vi "test_find_shift.vi"() -> ()   [LabVIEW 2016]
uses:
  <vilib>/Platform/TimedLoop/XDataNode/timing_clust.ctl
  <vilib>/Platform/TimedLoop/XDataNode/nitl_modes.ctl
  <vilib>/Platform/TimedLoop/XDataNode/wakeup.ctl
  <vilib>/platform/TimedLoop/XDataNode/XDataNode.xnode
  <vilib>/Platform/TimedLoop/XDataNode/XDNodeRunTimeDep.lvlib
panel:
  out "Ref Cropped":T1(plugin-control)
  out "ROI":T1(plugin-control)
  out "Y Pos":i32[](array[numeric])
  out "X Pos":i32[](array[numeric])
  out "Y Pos":i32[](graph)
  out "X Pos":i32[](graph)
  out "Surface Height":dbl[](graph)
  out "Y Shift":i32[](graph)
  out "X Shift":i32[](graph)
  out "Current Image":dbl=1000.0
  out "Surface Height":i32[](array[numeric])
  out "Y Shifts":i32[](array[numeric])
  out "X Shifts":i32[](array[numeric])
  in  "Vertical Search Range":dbl=50.0
  in  "ROI Horizontal Size":dbl=50.0
  in  "ROI Vertical Size":dbl=50.0
  in  "ROI Vertical Offset":dbl
  in  "Struc El Size":i32=10
  in  "Threshold Multiplier":sgl=2.0
  in  "Simulated FPS":dbl=50.0
  in  "stop":bool
  out "Num Images":dbl=1000.0
  in  "AVI File for Simulated Raw B Scan Images":path=path "C:/Users/Applied Optics Group/Desktop/DCF Paper Data Processing/data/2020_08_04_2dcheckerboard_AF/Large_grid/OCT_raw_vol.avi"
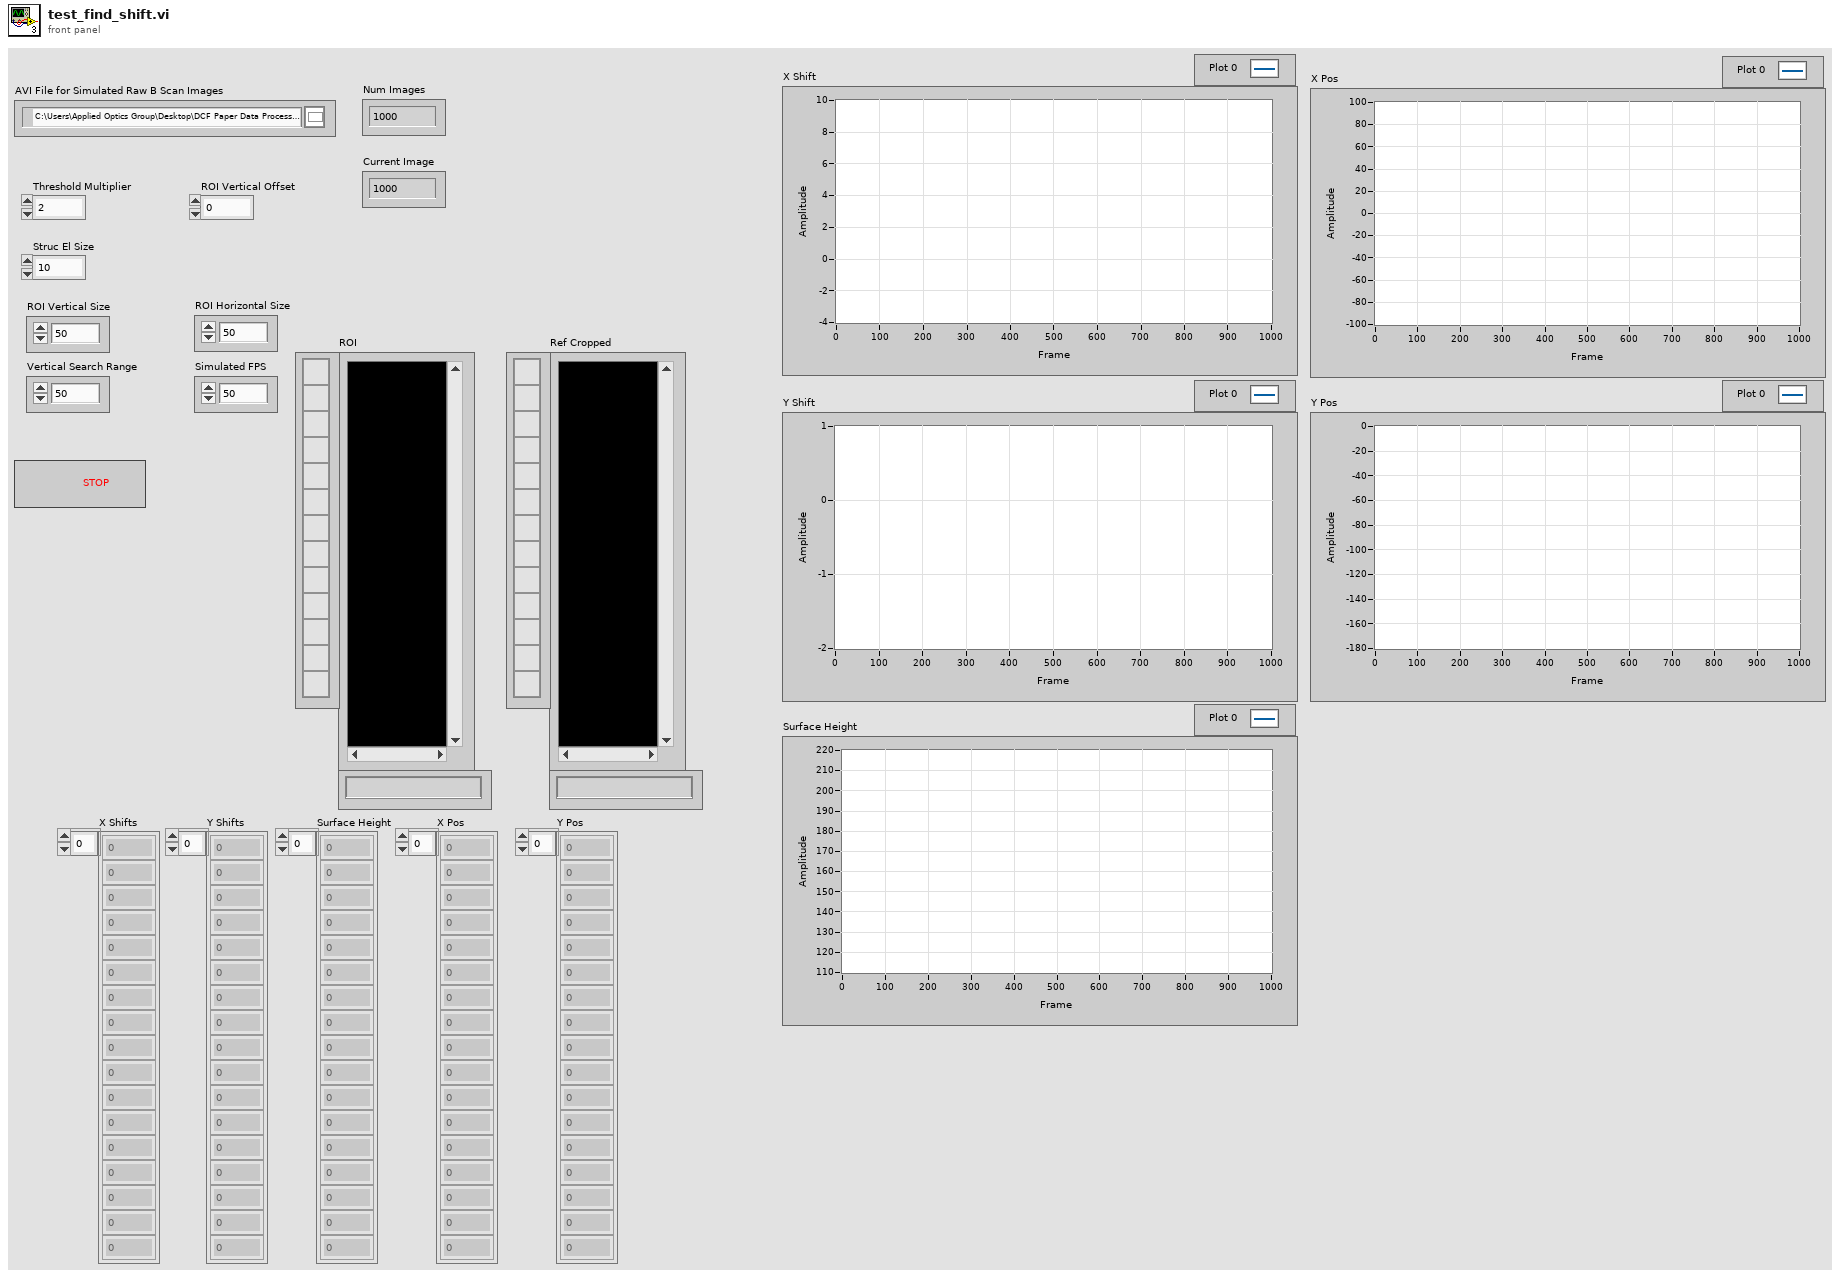
[diagram p1: front panel]
types:
  T1 = typedef "IMAQ Image.ctl" = refnum<image>
  T2 = typedef "Image Type" = u32
  T3 = typedef "XDNodeRunTimeDep.lvlib/timing_clust.ctl" = cluster{"Expected End [f-1]":u64, "Actual End [f-1]":u64, "Finished Late? [f-1]":bool, "Expected End [i-1]":u64, "Actual End [i-1]":u64, "Finished Late? [i-1]":bool, "Expected Start [i]":u64, "Actual Start [i]":u64, "Expected Start [f]":u64, "Actual Start [f]":u64, "Source Name":string, "Structure Name":string, "Period":i64, "Deadline":i64, "Offset":i64, "Start":i64, "Priority":i32, "Timeout":i32, "Mode":T4, "Wakeup Reason":T5, "Error":errorcluster, "Source Type":string, "Secondary Source Type":string, "Global End Time":u64, "Global Start Time":u64, "Frame Duration":u64, "Iteration Duration":u64, "Assigned CPU":i32, "I/O Scan Engine Mode":u32}
  T4 = typedef "XDNodeRunTimeDep.lvlib/nitl_modes.ctl" = enum32{"No Change", "Process missed periods, maintain original phase", "Discard missed periods, maintain original phase", "Process missed periods, ignore original phase", "Discard missed periods, ignore original phase"}
  T5 = typedef "XDNodeRunTimeDep.lvlib/wakeup.ctl" = enum32{"Normal", "Aborted", "Asynchronous wakeup", "Timing source error", "Timed loop error", "Timeout"}
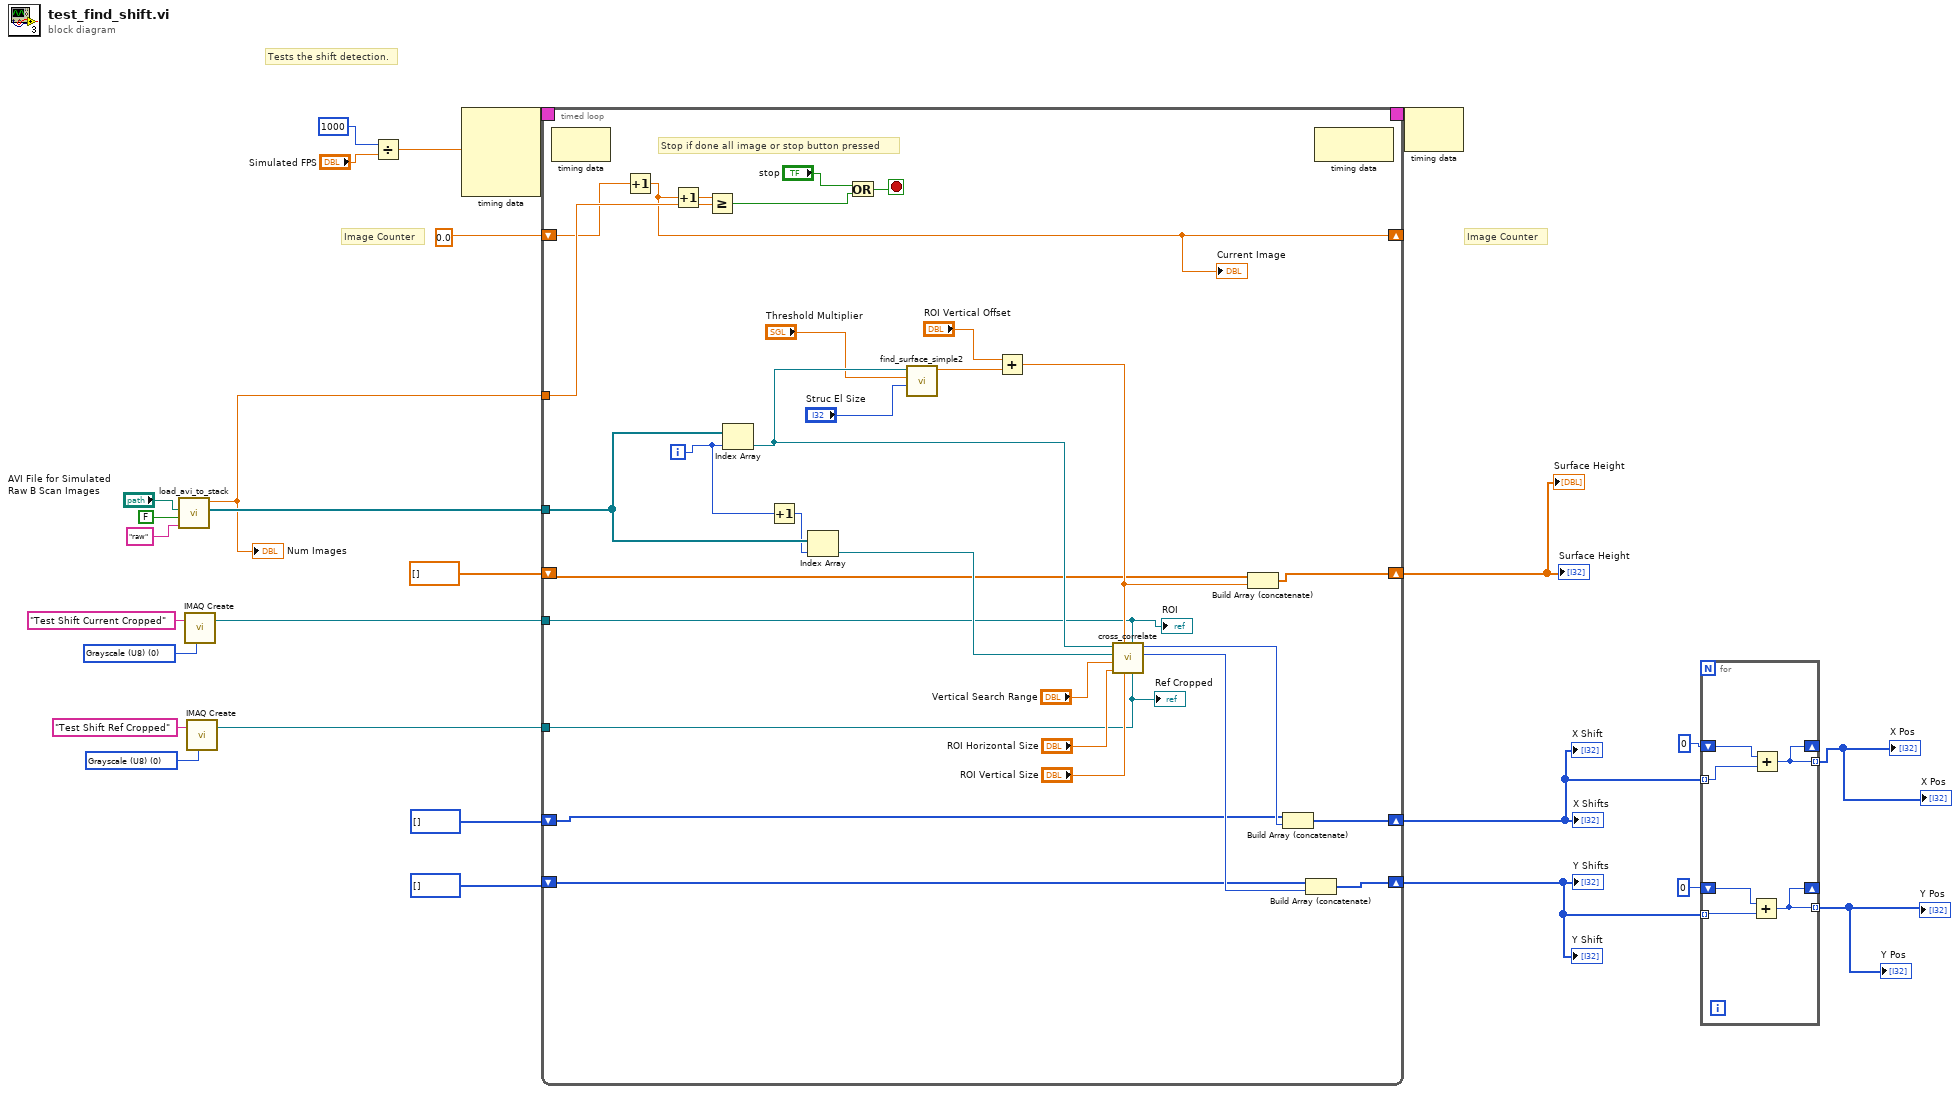
[diagram p0: block diagram]
diagram:
  w15 = T2 0 items=["Grayscale (U8)", "Grayscale (I16)", "Grayscale (SGL)", "Complex (CSG)", "RGB (U32)", "HSL (U32)", "RGB (U64)", "Grayscale (U16)"] ("Image Type")
  w17 = T2 0 items=["Grayscale (U8)", "Grayscale (I16)", "Grayscale (SGL)", "Complex (CSG)", "RGB (U32)", "HSL (U32)", "RGB (U64)", "Grayscale (U16)"] ("Image Type")
  # "Tests the shift detection."
  # "Image Counter"
  # "Image Counter"
  n1 = call "load_avi_to_stack.vi"("Image Prefix"="raw", "Preview"=FALSE, "AVI File"="AVI File for Simulated Raw B Scan Images") -> ("Image Array"=w24:T1[], "Num Images"=w11:dbl)  [unwired: 7 in]
  "Num Images" <- w11
  n2 = call "IMAQ Create"("Image Name"="Test Shift Current Cropped", "Image Type"=w17) -> ("New Image"=w16:T1)  [unwired: 3 in, 1 out]
  n3 = call "IMAQ Create"("Image Name"="Test Shift Ref Cropped", "Image Type"=w15) -> ("New Image"=w13:T1)  [unwired: 3 in, 1 out]
  n4 = Divide(x=1000, y="Simulated FPS") -> (x/y=w19:dbl)
  n5 = node-c288(w19) -> (w23:T3)  [unwired: 3 in]
  n6 = timed-loop {
    tunnel: w24 -> [w55]
    timing: w23 -> [_]
    timing-out: [_] -> w22
    tunnel: w16 -> [w29]
    tunnel: w13 -> [w28]
    tunnel: w11 -> [w57]
    shift-right: [w30] -> _
    shift-left: sgl 0.0 ("Pixel Value (U8, U16, I16, Float)") -> [w31]
    shift-right: [w38] -> w5
    shift-left: i32[] [] -> [w39]
    shift-right: [w40] -> w6
    shift-left: i32[] [] -> [w41]
    shift-right: [w33] -> w7
    shift-left: dbl[] [] -> [w32]
    i -> [w54]
    stop <- w37 stop-if-true
    # "Stop if done all image or stop button pressed"
    n7 = node-c288() -> ()  [unwired: 1 in, 1 out]
    n8 = Increment(x=w31) -> (x+1=w30:sgl)
    "Current Image" <- w30
    n9 = Increment(x=w30) -> (x+1=w56:sgl)
    n10 = Greater Or Equal?(x=w56, y=w57) -> (x >= y?=w35:bool)
    n11 = Index Array(array=w55, index=w54) -> (element=w51:T1)
    n12 = Increment(x=w54) -> (x+1=w53:i32)
    n13 = Index Array(array=w55, index=w53) -> (element=w52:T1)
    n14 = Or(x="stop", y=w35) -> (x .or. y?=w37:bool)
    n15 = call "find_surface_simple2.vi"("Struc El Size"="Struc El Size", "Threshold Multiplier"="Threshold Multiplier", "Image In"=w51) -> ("average surface height"=w48:dbl)  [unwired: 7 in, 1 out]
    n16 = Add(x="ROI Vertical Offset", y=w48) -> (x+y=w34:dbl)
    n17 = call "cross_correlate.vi"("Ref Image Cropped"=w28, "Template Image Cropped"=w29, "Template Height"="ROI Vertical Size", "Depth"=w34, "Template Width"="ROI Horizontal Size", "Vertical Search Range"="Vertical Search Range", "Ref Image"=w52, "Template Image"=w51) -> ("y shift"=w42:i32, "x shift"=w43:i32)  [unwired: 2 out]
    n18 = Build Array (concatenate)(w32, w34) -> (w33:dbl[])
    n19 = Build Array (concatenate)(w41, w43) -> (w40:i32[])
    n20 = Build Array (concatenate)(w39, w42) -> (w38:i32[])
    n21 = node-c288() -> ()  [unwired: 1 in, 1 out]
    "ROI" <- w29
    "Ref Cropped" <- w28
  }
  "X Shifts" <- w6
  "Y Shifts" <- w5
  "Surface Height" <- w7
  "X Shift" <- w6
  "Y Shift" <- w5
  "Surface Height" <- w7
  n22 = node-c288(w22) -> ()  [unwired: 1 out]
  n23 = for {
    tunnel: w6 -> [w65] mode=indexing
    tunnel: w5 -> [w63] mode=indexing
    shift-right: [w61] -> _
    shift-left: 0 -> [w64]
    shift-right: [w60] -> _
    shift-left: 0 -> [w62]
    tunnel: [w61] -> w2 mode=indexing
    tunnel: [w60] -> w1 mode=indexing
    n24 = Add(x=w62, y=w63) -> (x+y=w60:i32)
    n25 = Add(x=w64, y=w65) -> (x+y=w61:i32)
  }
  "X Pos" <- w2
  "Y Pos" <- w1
  "X Pos" <- w2
  "Y Pos" <- w1
